vi "Dye Recipe Table Step by Index.vi"(8 "error in (no error)":errorcluster, 9 "Dye Color":u32(colorbox), 10 "Index":u64, 11 "Kitchen Messaging Interface in":refnum<class "Kitchen Messaging Interface.lvclass">) -> (0 "error out":errorcluster, 3 "Kitchen Messaging Interface out":refnum<class "Kitchen Messaging Interface.lvclass">)   [LabVIEW 2024, in "Kitchen Messaging Interface.lvlib" / "Kitchen Messaging Interface.lvclass"]
uses:
  Kitchen Messaging Interface.lvclass
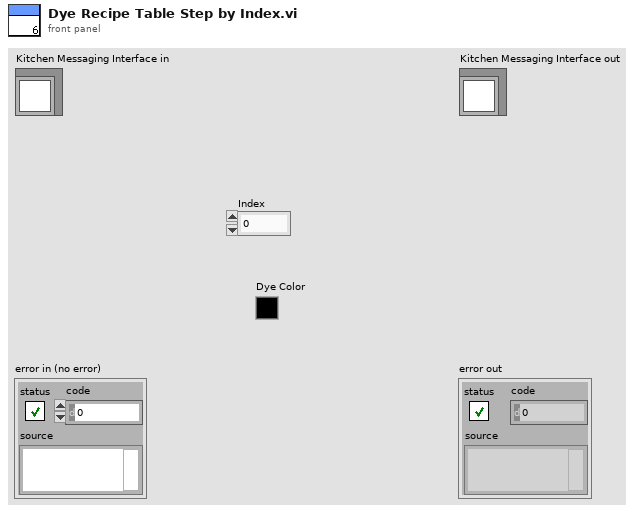
[diagram p1: front panel]
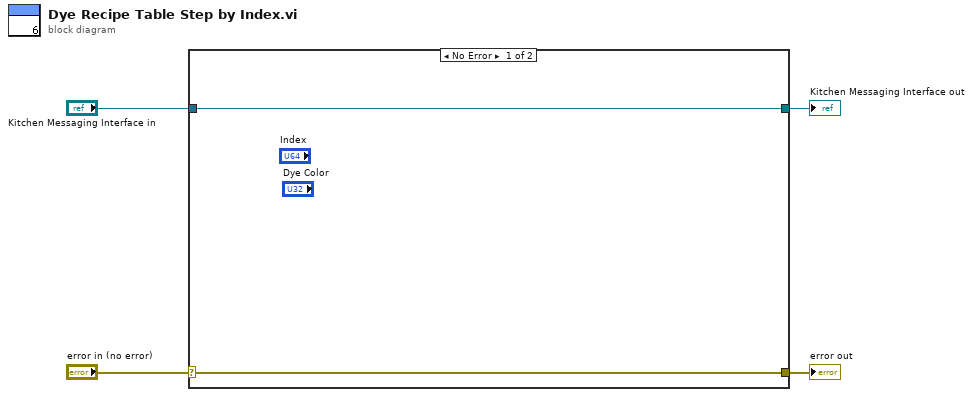
[diagram p0: block diagram]
diagram:
  n1 = case shown="No Error" "error in (no error)" {
    selector: "error in (no error)" -> [w5 w8]
    tunnel: [w5 w8] -> w3
    tunnel: [w6 w7] -> w1
    tunnel: "Kitchen Messaging Interface in" -> [w6 w7]
    frame No Error {
    }
    frame Error {
    }
  }
  "error out" <- w3
  "Kitchen Messaging Interface out" <- w1
